vi "Get Default VeriStand Application Path.vi"(8 "error in (no error)":errorcluster) -> (0 "error out":errorcluster, 3 "Default VeriStand App Path":path)   [LabVIEW 2015, in "ni-veristand-steps-runtime-lib.lvlib"]
uses:
  ni-veristand-steps-runtime-lib.lvlib
  <vilib>/Utility/sysdir.llb/System Directory Type.ctl
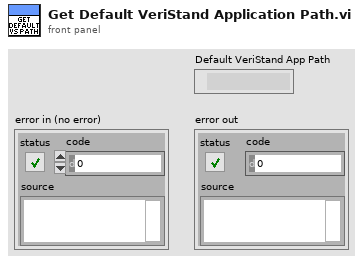
[diagram p1: front panel]
types:
  T1 = typedef "System Directory Type.ctl" = i32
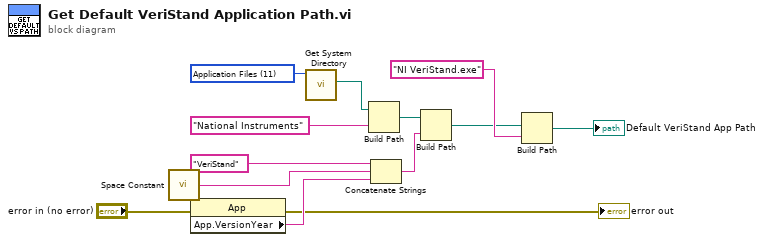
[diagram p0: block diagram]
diagram:
  w13 = T1 11 items=["User Home"=0, "User Desktop"=1, "User Documents"=2, "User Application Data"=3, "User Preferences"=4, "User Temporary"=5, "Public Documents"=6, "Public Application Data"=7, "Public Preferences"=8, "Public Cache"=13, "System Core Libraries"=9, "System Installed Libraries"=10, "Application Files"=11, "Boot Volume Root"=12] ("system directory type")
  n1 = call <vilib>:"Space Constant.vi"() -> ("String"=w9:string)
  n2 = property class="App"(error in="error in (no error)") -> (error out=→"error out":errorcluster, "App.VersionYear"=w8:string)  [unwired: 1 in, 1 out]
  n3 = call <vilib>:"Get System Directory.vi"("system directory type"=w13) -> ("system directory"=w4:path)  [unwired: 10 in]
  n4 = Build Path(base path=w4, name or relative path="National Instruments") -> (appended path=w6:path)
  n5 = Concatenate Strings("VeriStand" ("name or relative path"), w9, w8) -> (w10:string)
  n6 = Build Path(base path=w6, name or relative path=w10) -> (appended path=w11:path)
  n7 = Build Path(base path=w11, name or relative path="NI VeriStand.exe") -> (appended path=→"Default VeriStand App Path":path)
